vi "ADIS16448_RoboRIO_Teensy_Open.vi"(7 "error in":errorcluster, 9 "Z Orientation":enum16{"Z Up", "Z Down"}(ring)=enum."Z Down") -> (0 "error out":errorcluster, 3 "SerialPortRef":T1)   [LabVIEW 2016, in "RoboRIO-Teensy-ADIS16448-Interface.lvlib"]
uses:
  RoboRIO-Teensy-ADIS16448-Interface.lvlib
  <vilib>/Rock Robotics/WPI/SerialPort/WPI_SerialPortRef.ctl
  <vilib>/Rock Robotics/WPI/SerialPort/WPI_SerialPort.ctl
  ADIS16448_RoboRIO_Teensy_Loop.vi
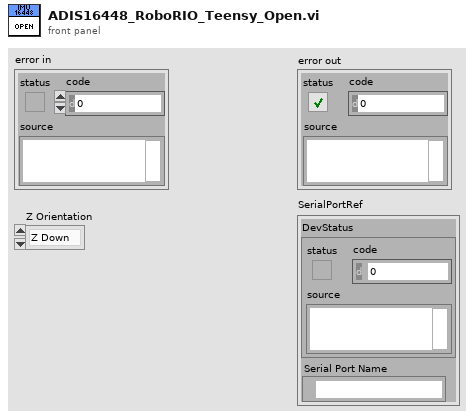
[diagram p1: front panel]
types:
  T1 = typedef "WPI_SerialPortRef.ctl" = cluster{"DevStatus":errorcluster, "Serial Port Name":refnum<visa-resource-name>}
  T2 = typedef "WPI_SerialPort.ctl" = enum16{"Onboard RS-232", "MXP TTL", "USB 1", "USB 2"}
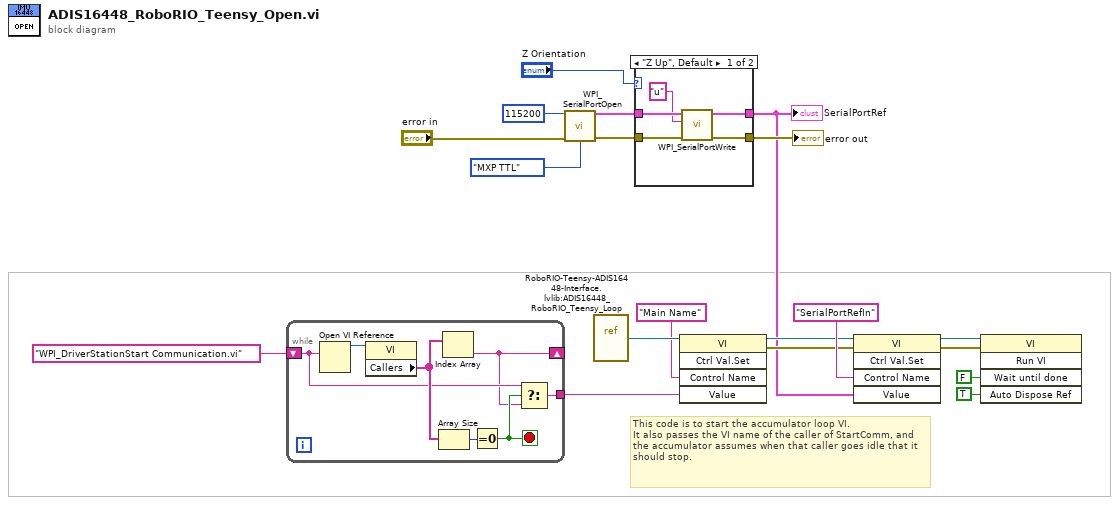
[diagram p0: block diagram]
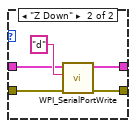
[diagram p2: hidden frame]
diagram:
  # "This code is to start the accumulator loop VI.\nIt also passes the VI name of the caller of StartComm, and the accumulator assumes when that caller goes idle that it should stop."
  n1 = while {
    shift-right: [w21] -> _
    shift-left: "WPI_DriverStationStart Communication.vi" -> [w22]
    tunnel: [w20] -> w3
    stop <- w23 stop-if-true
    n2 = Open VI Reference(vi path=w22) -> (vi reference=w26:refnum<vi>)  [unwired: 1 in, 5 out]
    n3 = property class="VI"(reference=w26) -> ("Callers"=w24:string[])  [unwired: 1 in, 2 out]
    n4 = Array Size(array=w24) -> (size(s)=w25:i32)
    n5 = Index Array(array=w24) -> (element=w21:string)  [unwired: 1 in]
    n6 = Equal To 0?(x=w25) -> (x = 0?=w23:bool)
    n7 = Select(t=w22, s=w23, f=w21) -> (s? t:f=w20:string)
  }
  n8 = call <vilib>:"WPI_SerialPortOpen.vi"("Baud Rate"=u32 115200, "error in (no error)"="error in", "Serial Port"=WPI_SerialPort."MXP TTL") -> ("SerialPortRef"=w16:T1, "error out"=w15:errorcluster)  [unwired: 11 in]
  n9 = vi-ref "RoboRIO-Teensy-ADIS16448-Interface.lvlib:ADIS16448_RoboRIO_Teensy_Loop.vi"() -> (w5:refnum<vi>)
  n10 = case shown="\"Z Up\", Default" "Z Orientation" {
    tunnel: w16 -> [w31 w35]
    tunnel: w15 -> [w30 w34]
    tunnel: [w29 w33] -> w1
    tunnel: [w28 w32] -> w14
    frame "Z Up", Default {
      n11 = call <vilib>:"WPI_SerialPortWrite.vi"("error in (no error)"=w30, "Buffer"="u", "SerialPortRef"=w31) -> ("error out"=w28:errorcluster, "SerialPortRef"=w29:T1)  [unwired: 6 in, 1 out]
    }
    frame "Z Down" {
      n12 = call <vilib>:"WPI_SerialPortWrite.vi"("error in (no error)"=w34, "Buffer"="d", "SerialPortRef"=w35) -> ("error out"=w32:errorcluster, "SerialPortRef"=w33:T1)  [unwired: 6 in, 1 out]
    }
  }
  "error out" <- w14
  "SerialPortRef" <- w1
  n13 = invoke class="VI" method="Ctrl Val.Set"(reference=w5, "Control Name"="Main Name", "Value"=w3) -> (reference out=w2:refnum<vi>, error out=w7:errorcluster)  [unwired: 2 in, 3 out]
  n14 = invoke class="VI" method="Ctrl Val.Set"(reference=w2, error in=w7, "Control Name"="SerialPortRefIn", "Value"=w1) -> (reference out=w12:refnum<vi>, error out=w8:errorcluster)  [unwired: 1 in, 3 out]
  n15 = invoke class="VI" method="Run VI"(reference=w12, error in=w8, "Wait until done"=FALSE ("Wait Until Done"), "Auto Dispose Ref"=TRUE ("Auto Dispose Reference")) -> ()  [unwired: 1 in, 5 out]
